vi "读写键断.vi"(7 "枚举":enum16{"write", "read", "读键", "读段", ""}(ring), 8 "写入值":string caption="值", 9 "键":string, 10 "段":string, 11 "创建文件路径":path=path "D:/Labviewprogram/多账户登录") -> (0 "读取的值":string caption="值", 1 "键名":string[](array[string]), 2 "段名":string[](array[string]))   [LabVIEW 2018]
uses:
  <vilib>/Utility/config.llb/Write Key (String).vi
  <vilib>/Utility/config.llb/Read Key (String).vi
  <vilib>/Utility/config.llb/NI_LVConfig.lvlib
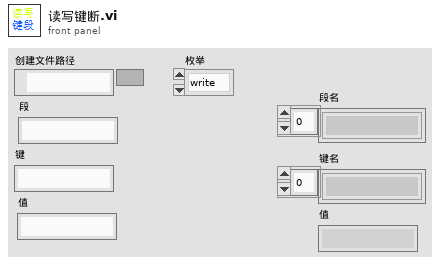
[diagram p1: front panel]
types:
  T1 = typedef "NI_LVConfig.lvlib/Config Data RefNum.ctl" = refnum<k1>
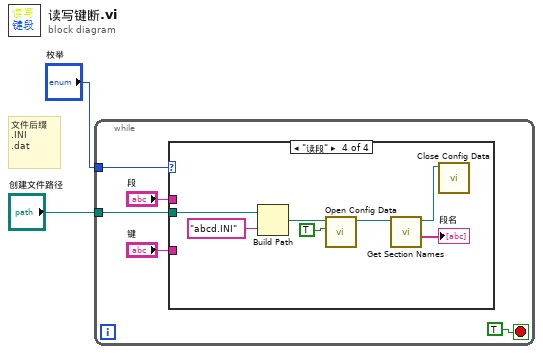
[diagram p0: block diagram]
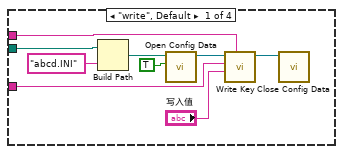
[diagram p2: hidden frame]
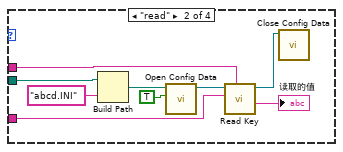
[diagram p3: hidden frame]
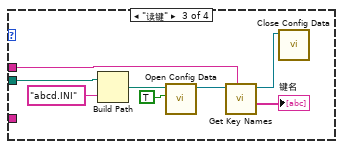
[diagram p4: hidden frame]
diagram:
  # "文件后缀\n.INI\n.dat"
  n1 = while {
    tunnel: "枚举" -> [w6]
    tunnel: "创建文件路径" -> [w5]
    stop <- TRUE stop-if-true
    n2 = case shown="\"读段\"" w6 {
      tunnel: w5 -> [w10 w22 w28 w35]
      tunnel: "段" -> [w8 w20 w27 _]
      tunnel: "键" -> [w9 w19 _ _]
      frame "write", Default {
        n3 = Build Path(base path=w10, name or relative path="abcd.INI" ("名称或相对路径")) -> (appended path=w15:path)
        n4 = call <vilib>:"Open Config Data.vi"("create file if necessary (T)"=TRUE, "configuration file path"=w15) -> ("refnum"=w14:T1)  [unwired: 7 in, 2 out]
        n5 = call-poly <vilib>:"Write Key.vi"("section"=w8, "value"="写入值", "key"=w9, "refnum"=w14) -> ("refnum out"=w13:T1)  [unwired: 5 in, 2 out]
        n6 = call <vilib>:"Close Config Data.vi"("refnum"=w13) -> ()  [unwired: 9 in, 2 out]
      }
      frame "read" {
        n7 = Build Path(base path=w22, name or relative path="abcd.INI" ("名称或相对路径")) -> (appended path=w25:path)
        n8 = call <vilib>:"Open Config Data.vi"("create file if necessary (T)"=TRUE, "configuration file path"=w25) -> ("refnum"=w21:T1)  [unwired: 7 in, 2 out]
        n9 = call-poly <vilib>:"Read Key.vi"("section"=w20, "key"=w19, "refnum"=w21) -> ("value"=→"读取的值":string, "refnum out"=w18:T1)  [unwired: 5 in, 2 out]
        n10 = call <vilib>:"Close Config Data.vi"("refnum"=w18) -> ()  [unwired: 9 in, 2 out]
      }
      frame "读键" {
        n11 = Build Path(base path=w28, name or relative path="abcd.INI" ("名称或相对路径")) -> (appended path=w33:path)
        n12 = call <vilib>:"Open Config Data.vi"("create file if necessary (T)"=TRUE, "configuration file path"=w33) -> ("refnum"=w30:T1)  [unwired: 7 in, 2 out]
        n13 = call <vilib>:"Get Key Names.vi"("section"=w27, "refnum"=w30) -> ("key names"=→"键名":string[], "refnum out"=w29:T1)  [unwired: 6 in, 2 out]
        n14 = call <vilib>:"Close Config Data.vi"("refnum"=w29) -> ()  [unwired: 9 in, 2 out]
      }
      frame "读段" {
        n15 = Build Path(base path=w35, name or relative path="abcd.INI" ("名称或相对路径")) -> (appended path=w40:path)
        n16 = call <vilib>:"Open Config Data.vi"("create file if necessary (T)"=TRUE, "configuration file path"=w40) -> ("refnum"=w39:T1)  [unwired: 7 in, 2 out]
        n17 = call <vilib>:"Get Section Names.vi"("refnum"=w39) -> ("section names"=→"段名":string[], "refnum out"=w38:T1)  [unwired: 8 in, 1 out]
        n18 = call <vilib>:"Close Config Data.vi"("refnum"=w38) -> ()  [unwired: 9 in, 2 out]
      }
    }
  }
